vi "Read Temperature.vi"(8 "Error In":errorcluster, 9 "Thermocouple #":u8, 10 "Port":i8, 11 "FPGA VI Reference In":T1) -> (0 "error out":errorcluster, 2 "Temperature Out (C)":fxp<+,12,10>, 3 "FPGA VI Reference Out":T1)   [LabVIEW 2014]
uses:
  Controls/FPGA Reference.ctl
  Controls/SPI Configuration Cluster.ctl
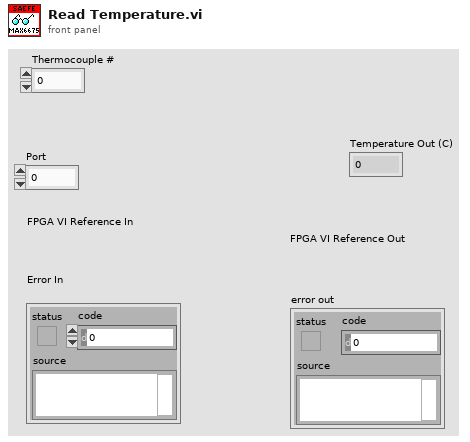
[diagram p1: front panel]
types:
  T1 = typedef "FPGA Reference.ctl" = refnum<k20>
  T2 = typedef "SPI Configuration Cluster.ctl" = cluster{"CS":u8, "Clock Rate (Hz)":dbl, "Clock Mode":u8, "CS Active State":bool}
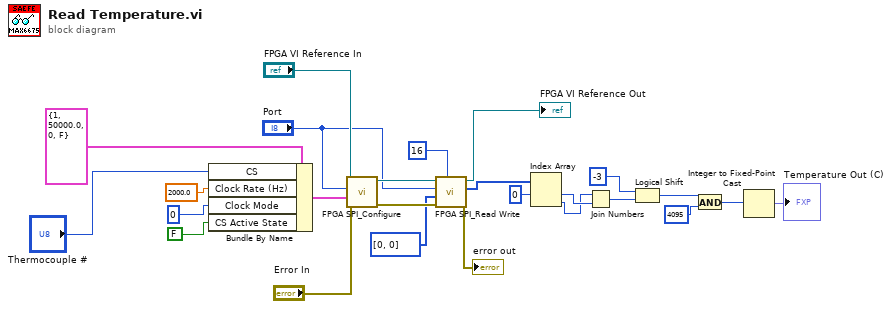
[diagram p0: block diagram]
diagram:
  n1 = Bundle By Name(cluster=T2 {"CS"=1, "Clock Rate (Hz)"=50000.0, "Clock Mode"=0, "CS Active State"=FALSE} ("Configuration Cluster"), "CS"="Thermocouple #", "Clock Rate (Hz)"=2000.0, "Clock Mode"=u8 0, "CS Active State"=FALSE) -> (w21:T2)
  n2 = call "FPGA SPI_Configure.vi"("error in"="Error In", "Configuration Cluster"=w21, "Port"="Port", "FPGA VI Reference"="FPGA VI Reference In") -> ("error out"=w17:errorcluster, "FPGA VI Reference Out"=w18:T1)  [unwired: 5 in, 1 out]
  n3 = call "FPGA SPI_Read Write.vi"("Total Bits"=u16 16, "error in"=w17, "Write Data"=u8[] [0, 0], "Port"="Port", "FPGA VI Reference"=w18) -> ("error out"=→"error out":errorcluster, "Read Data"=w11:u8[], "FPGA VI Reference Out"=→"FPGA VI Reference Out":T1)  [unwired: 4 in]
  n4 = Index Array(array=w11, index #1=0 ("index")) -> (element #1=w9:u8, element #2=w8:u8)  [unwired: 1 in]
  n5 = Join Numbers(hi=w8, lo=w9) -> ((hi.lo)=w7:u16)
  n6 = Logical Shift(y=i16 -3, x=w7) -> (x << y=w5:u16)
  n7 = And(x=w5, y=u16 4095) -> (x .and. y?=w3:u16)
  n8 = Integer to Fixed-Point Cast(integer=w3) -> (fixed-point=→"Temperature Out (C)":fxp<+,12,10>)  [unwired: 1 in]
